vi "write_attributes.vi"(8 "error in (no error)":errorcluster, 10 "attributes":T1, 11 "BayesianGaussianMixture in":refnum<class "BayesianGaussianMixture.lvclass">) -> (0 "error out":errorcluster, 3 "BayesianGaussianMixture out":refnum<class "BayesianGaussianMixture.lvclass">)   [LabVIEW 2020, in "BayesianGaussianMixture.lvclass"]
uses:
  BayesianGaussianMixture.lvclass
  Controls/bayesian_gaussian_mixture_attributes.ctl
  BayesianGaussianMixture.lvclass/BayesianGaussianMixture.ctl
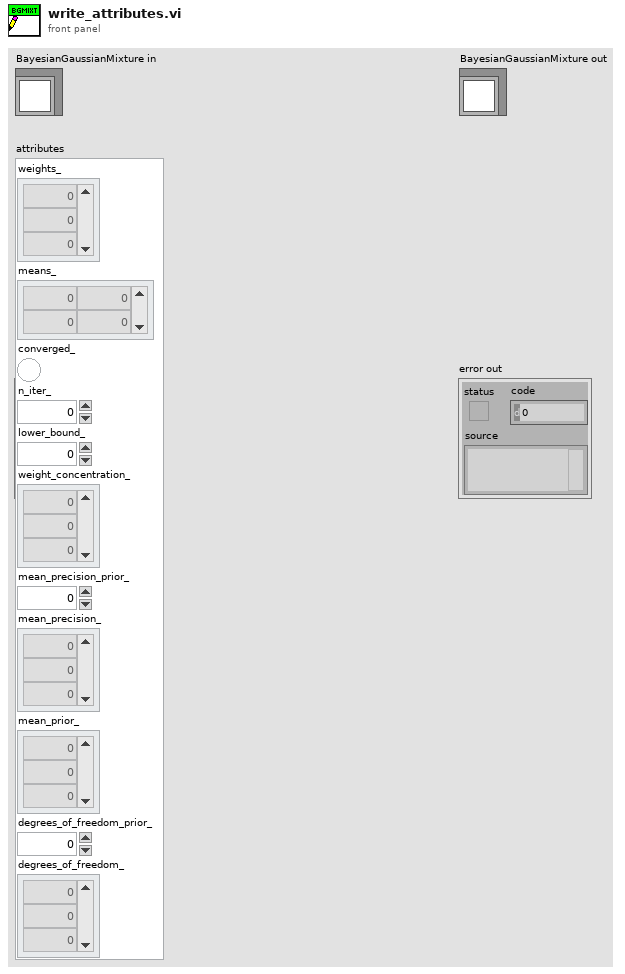
[diagram p1: front panel]
types:
  T1 = typedef "bayesian_gaussian_mixture_attributes.ctl" = cluster{"weights_":dbl[], "means_":dbl[][], "converged_":bool, "n_iter_":dbl, "lower_bound_":dbl, "weight_concentration_":dbl[][], "mean_precision_prior_":dbl, "mean_precision_":dbl[], "mean_prior_":dbl[], "degrees_of_freedom_prior_":dbl, "degrees_of_freedom_":dbl[]}
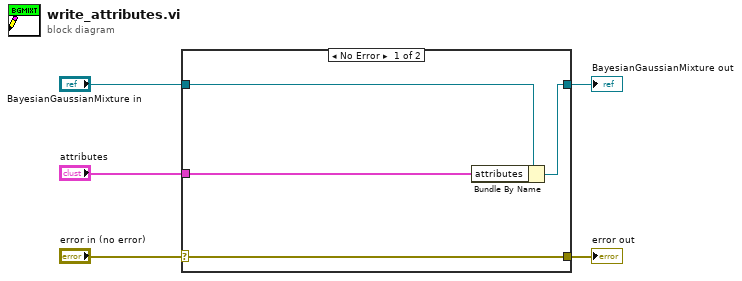
[diagram p0: block diagram]
diagram:
  n1 = case shown="No Error" "error in (no error)" {
    selector: "error in (no error)" -> [w9 w10]
    tunnel: [w9 w10] -> w4
    tunnel: [w7 w11] -> w2
    tunnel: "BayesianGaussianMixture in" -> [w8 w11]
    tunnel: "attributes" -> [w6 _]
    frame No Error {
      n2 = Bundle By Name(cluster=w8, "attributes"=w6) -> (w7:refnum<class "BayesianGaussianMixture.lvclass">)
    }
    frame Error {
    }
  }
  "error out" <- w4
  "BayesianGaussianMixture out" <- w2
